vi "Simple_traffic_light_demo.vi"() -> ()   [LabVIEW 2019]
panel:
  out "Green":bool
  out "Yellow":bool
  out "Red":bool
  in  "Frequency":dbl=10.1
  in  "Amplitude":dbl=1.0
  out "Waveform Chart":dynamicdata(graph)
  in  "stop":bool
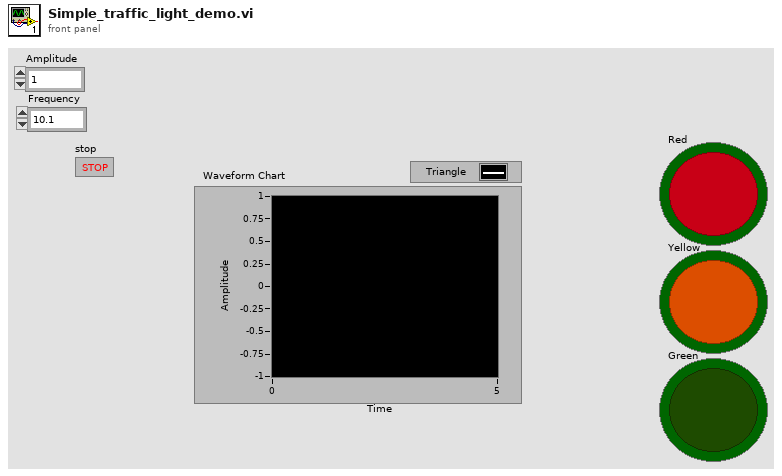
[diagram p1: front panel]
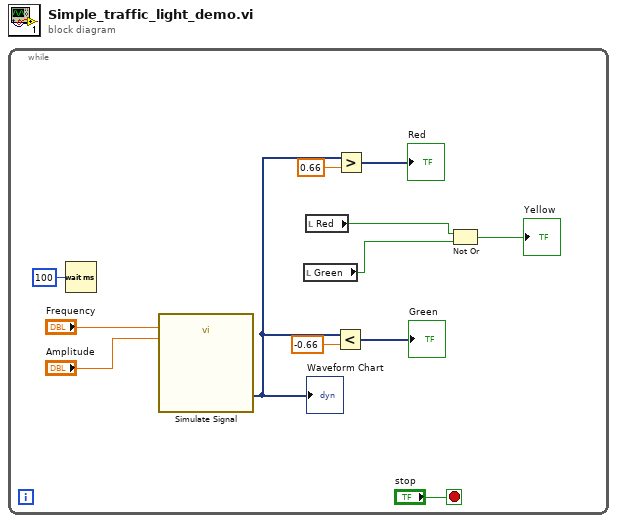
[diagram p0: block diagram]
diagram:
  n1 = while {
    stop <- "stop" stop-if-true
    n2 = Wait (ms)(milliseconds to wait=u32 100) -> ()  [unwired: 1 out]
    n3 = call "Simulate Signal"("Frequency"="Frequency", "Amplitude"="Amplitude") -> ("Triangle"=w6:dynamicdata)  [unwired: 12 in, 1 out]
    "Waveform Chart" <- w6
    n4 = local read "Green"() -> (w2:bool)
    n5 = local read "Red"() -> (w3:bool)
    n6 = Less?(x=w6, y=-0.66) -> (x < y?=→"Green":dynamicdata)
    n7 = Greater?(x=w6, y=0.66) -> (0:→"Red":dynamicdata)
    n8 = Not Or(1:w2, 2:w3) -> (0:→"Yellow":bool)
  }
